vi "Find_usb_com_port.vi"(8 "error in (no error)":errorcluster, 11 "USB search key":string="USB\\VID_1BC7*PID_1010*MI_02* ") -> (0 "error out":errorcluster, 2 "Found com port":bool, 3 "Comport":string)   [LabVIEW 2013]
panel:
  out "standard output":string="No matching devices found.\r\n"
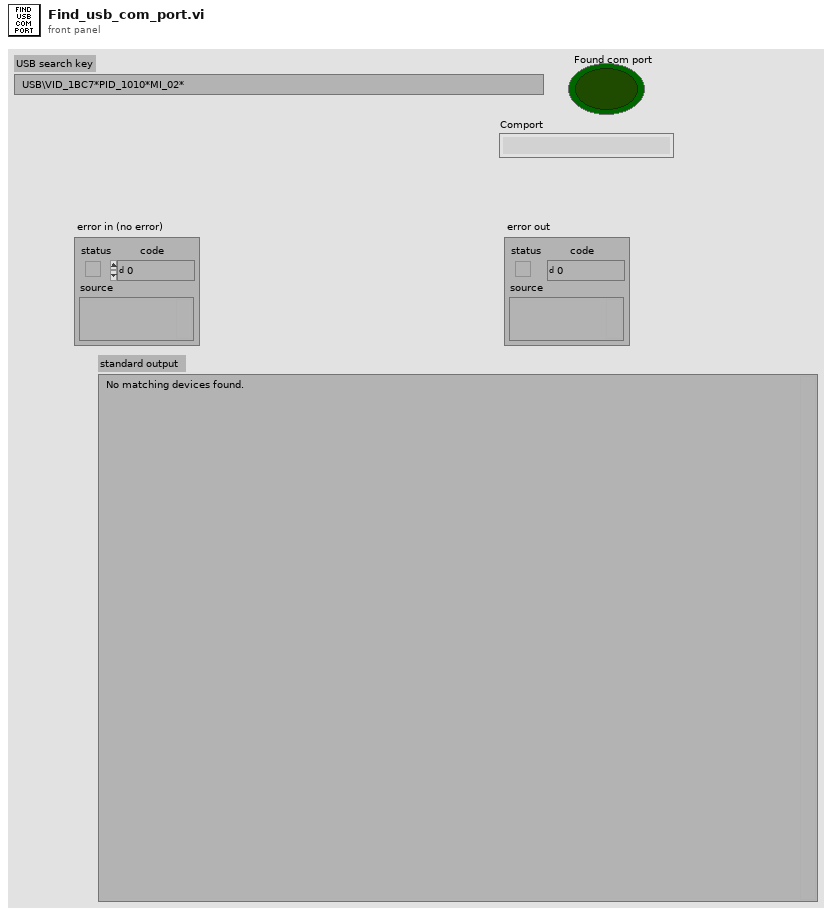
[diagram p1: front panel]
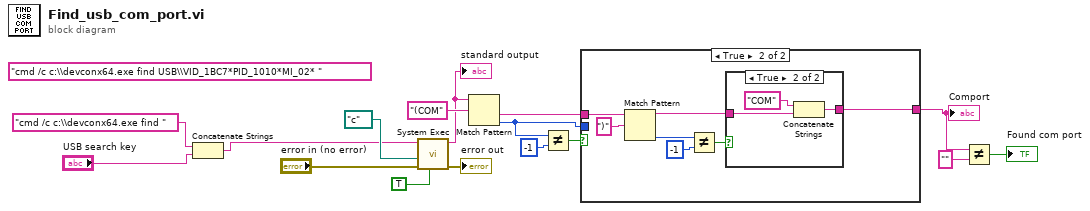
[diagram p0: block diagram]
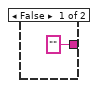
[diagram p2: hidden frame]
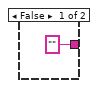
[diagram p3: hidden frame]
diagram:
  (unwired) "cmd /c c:\\devconx64.exe find USB\\VID_1BC7*PID_1010*MI_02* " ("command line")
  n1 = Concatenate Strings("cmd /c c:\\devconx64.exe find ", "USB search key") -> (w4:string)
  n2 = call <vilib>:"System Exec.vi"("run minimized? (F)"=TRUE, "error in (no error)"="error in (no error)", "working directory"=path "c:/", "command line"=w4) -> ("error out"=→"error out":errorcluster, "standard output"=w8:string)  [unwired: 4 in, 2 out]
  "standard output" <- w8
  n3 = Match Pattern(string=w8, regular expression="(COM") -> (after substring=w7:string, offset past match=w9:i32)  [unwired: 1 in, 2 out]
  n4 = Not Equal?(x=w9, y=-1) -> (x != y?=w10:bool)
  n5 = case shown="True" w10 {
    tunnel: w9 -> [_ _]
    tunnel: w7 -> [_ w20]
    tunnel: ["" ("standard output") w18] -> w3
    frame False {
    }
    frame True {
      n6 = Match Pattern(string=w20, regular expression=")") -> (before substring=w19:string, offset past match=w22:i32)  [unwired: 1 in, 2 out]
      n7 = Not Equal?(x=w22, y=-1) -> (x != y?=w21:bool)
      n8 = case shown="True" w21 {
        tunnel: ["" ("standard output") w26] -> w18
        tunnel: w19 -> [_ w27]
        frame False {
        }
        frame True {
          n9 = Concatenate Strings("COM" ("string"), w27) -> (w26:string)
        }
      }
    }
  }
  "Comport" <- w3
  n10 = Not Equal?(x=w3, y="") -> (x != y?=→"Found com port":bool)
